vi "generuj_nazwe_pliku.vi"(7 "Uwzględnij czas (F)":bool, 8 "error in (no error)":errorcluster, 9 "rozszerzenie":string, 10 "Nazwa bazowa":string, 11 "Application Directory":path) -> (0 "error out":errorcluster, 3 "appended path":path)   [LabVIEW 2014]
doc: "Generuje nazwę pliku do wczytania,\nz możliwością nadania czasu\nw formacie RRRR-MM-DD_GGMM"
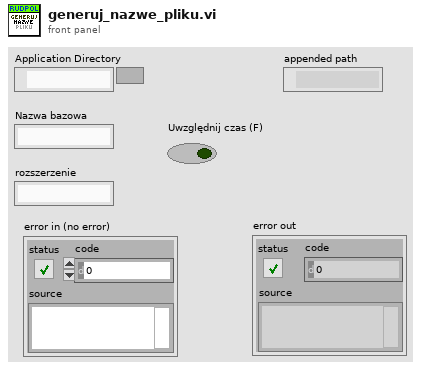
[diagram p1: front panel]
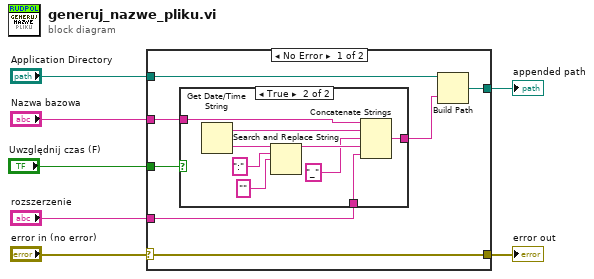
[diagram p0: block diagram]
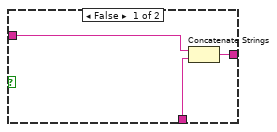
[diagram p2: hidden frame]
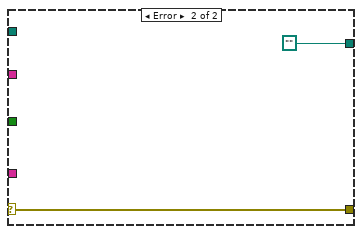
[diagram p3: hidden frame]
diagram:
  n1 = case shown="No Error" "error in (no error)" {
    selector: "error in (no error)" -> [w9 w28]
    tunnel: "rozszerzenie" -> [w14 _]
    tunnel: "Application Directory" -> [w13 _]
    tunnel: [w12 path ""] -> w5
    tunnel: "Nazwa bazowa" -> [w10 _]
    tunnel: [w9 w28] -> w2
    tunnel: "Uwzględnij czas (F)" -> [w8 _]
    frame No Error {
      n2 = case shown="True" w8 {
        tunnel: w14 -> [w16 w26]
        tunnel: [w17 w21] -> w11
        tunnel: w10 -> [w15 w18]
        frame False {
          n3 = Concatenate Strings(w15, w16) -> (w17:string)
        }
        frame True {
          n4 = Get Date/Time String() -> (date string=w19:string, time string=w22:string)  [unwired: 3 in]
          n5 = Search and Replace String(input string=w22, search string=":", replace string="" ("replace string (\"\")")) -> (result string=w25:string)  [unwired: 5 in, 3 out]
          n6 = Concatenate Strings(w18, w19, "_" ("string"), w25, w26) -> (w21:string)
        }
      }
      n7 = Build Path(base path=w13, name or relative path=w11) -> (appended path=w12:path)
    }
    frame Error {
    }
  }
  "appended path" <- w5
  "error out" <- w2
